vi "XML Script - Flat Sequence Structure.vi"(0 "x":i32=-1, 1 "y":i32=-1, 2 "out":i32=-1, 4 "frames (XML)":string, 6 "name":string, 9 "prefix (name)":string, 10 "in":i32=-1) -> (5 "name (wire source)":string, 7 "XML Script Command - Flat Sequence Structure":string)   [LabVIEW 2017]
uses:
  <vilib>/_script/XML Scripting/XML Script Tag.ctl
  <vilib>/_script/XML Scripting/XML Script Attribute.ctl
panel:
  # "position"
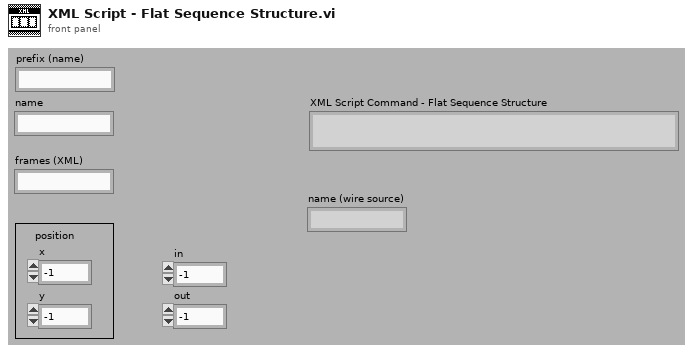
[diagram p1: front panel]
types:
  T1 = typedef "XML Script Attribute.ctl" = enum16{"name", "style", "path", "position", "in", "out", "width", "height", "index", "value", "default", "location", "offset", "typeindex", "size", "source", "destination", "indicator", "type", "controlname", "label", "conpaneidx", "mode", "description", "hasCondTerm", "linkIdentity", "caseselectortype", "concatInputs", "inName", "instantiationpath", "loopCondition", "IndexMode", "formulaInputs", "formulaOutputs", "msnFuncName", "msnIsDynamic", "msnIsODEUserFunction", "ignoreSearchDialog"}
  T2 = typedef "XML Script Tag.ctl" = enum16{"Script", "Function", "SubVI", "GrowableFunction", "Structure", "MultiframeStructure", "Frame", "Tunnel", "ShiftRegister", "Constant", "Control", "Terminal", "Wire", "StaticVIReference", "ControlTerminal", "CompoundArithmetic", "FlatSequence", "FlatSequenceFrame", "MathScriptCallByRef", "BuildArray", "GenericSubVI", "MathScriptNode"}
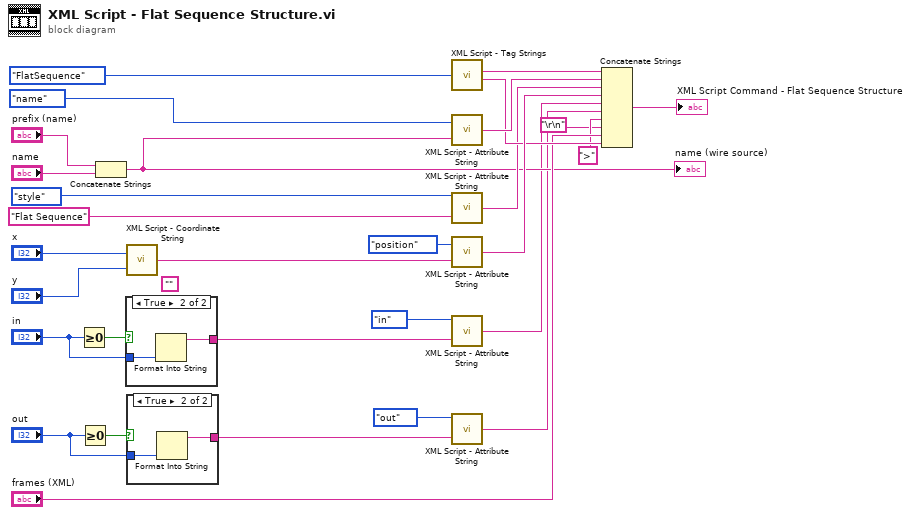
[diagram p0: block diagram]
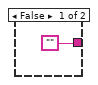
[diagram p2: hidden frame]
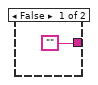
[diagram p3: hidden frame]
diagram:
  (unwired) ""
  n1 = Greater Or Equal To 0?(x="in") -> (x >= 0?=w4:bool)
  n2 = Greater Or Equal To 0?(x="out") -> (x >= 0?=w8:bool)
  n3 = Concatenate Strings("prefix (name)", "name") -> (w11:string)
  "name (wire source)" <- w11
  n4 = case shown="True" w4 {
    tunnel: "in" -> [_ w33]
    tunnel: ["" w32] -> w6
    frame False {
    }
    frame True {
      n5 = Format Into String(w33) -> (resulting string=w32:string)  [unwired: 3 in, 1 out]
    }
  }
  n6 = call <vilib>:"XML Script - Coordinate String.vi"("y"="y", "x"="x") -> ("(x,y)"=w21:string)
  n7 = case shown="True" w8 {
    tunnel: "out" -> [_ w36]
    tunnel: ["" w35] -> w10
    frame False {
    }
    frame True {
      n8 = Format Into String(w36) -> (resulting string=w35:string)  [unwired: 3 in, 1 out]
    }
  }
  n9 = call <vilib>:"XML Script - Tag Strings.vi"("XML Script Tag"=XML_Script_Tag."FlatSequence") -> ("XML String - Begin Tag"=w27:string, "XML String - End Tag"=w18:string)  [unwired: 2 in]
  n10 = call <vilib>:"XML Script - Attribute String.vi"("Attribute String"=w11, "XML Script Attribute"=XML_Script_Attribute."name") -> ("XML Script - Attribute String"=w24:string)
  n11 = call <vilib>:"XML Script - Attribute String.vi"("Attribute String"="Flat Sequence", "XML Script Attribute"=XML_Script_Attribute."style") -> ("XML Script - Attribute String"=w14:string)
  n12 = call <vilib>:"XML Script - Attribute String.vi"("Attribute String"=w21, "XML Script Attribute"=XML_Script_Attribute."position") -> ("XML Script - Attribute String"=w19:string)
  n13 = call <vilib>:"XML Script - Attribute String.vi"("Attribute String"=w6, "XML Script Attribute"=XML_Script_Attribute."in") -> ("XML Script - Attribute String"=w2:string)
  n14 = call <vilib>:"XML Script - Attribute String.vi"("Attribute String"=w10, "XML Script Attribute"=XML_Script_Attribute."out") -> ("XML Script - Attribute String"=w1:string)
  n15 = Concatenate Strings(w27, w24, w14, w19, w2, w1, ">" ("string"), "\r\n", "frames (XML)", w18) -> (→"XML Script Command - Flat Sequence Structure":string)
